vi "Update Values Buffer.vi"(8 "error in (no error)":errorcluster, 9 "buffer data":T1={"decimation"=0, "avg bandwidth"=0.0, "channels"=[], "byte order"=enum."little-endian", "buffer descriptor"={"buffer type"=enum."Engine", "plugin id"=0, "group id"=0, "transfer id"=0, "offset"=0, "length"=0}, "values channels"={"index"=0, "count"=0, "engine offset"=0}, "select start offset"=18446744073709551615, "select end offset"=0, "channel index"=-1} {"channels"."core"."string offset" format="%d bytes"; "avg bandwidth" format="%.0g bytes"}, 10 "buffer in":u8[](array[numeric]), 11 "values buffer in":u8[](array[numeric])) -> (0 "error out":errorcluster, 2 "buffer out":u8[](array[numeric]), 3 "values buffer out":u8[](array[numeric]))   [LabVIEW 2017, in "DSF Core.lvlib"]
uses:
  DSF Core.lvlib
  Buffer Reader/Buffer Data.ctl
  Typedefs/DSF Engine Channel Configuration.ctl
  Typedefs/Core Channel Configuration.ctl
  Typedefs/DSF Data Type.ctl
  Typedefs/DSF Settings Info.ctl
  Typedefs/DSF Version Info.ctl
  Typedefs/DSF Byte Order.ctl
  Classes/Thread/Data Server/DSF Buffer Subset Descriptor.ctl
  Typedefs/DSF Buffer Type.ctl
  Values Channels.ctl
  Classes/Framework/Framework.lvclass
  Classes/Configuration/Base/Channel/Channel Configuration.lvclass
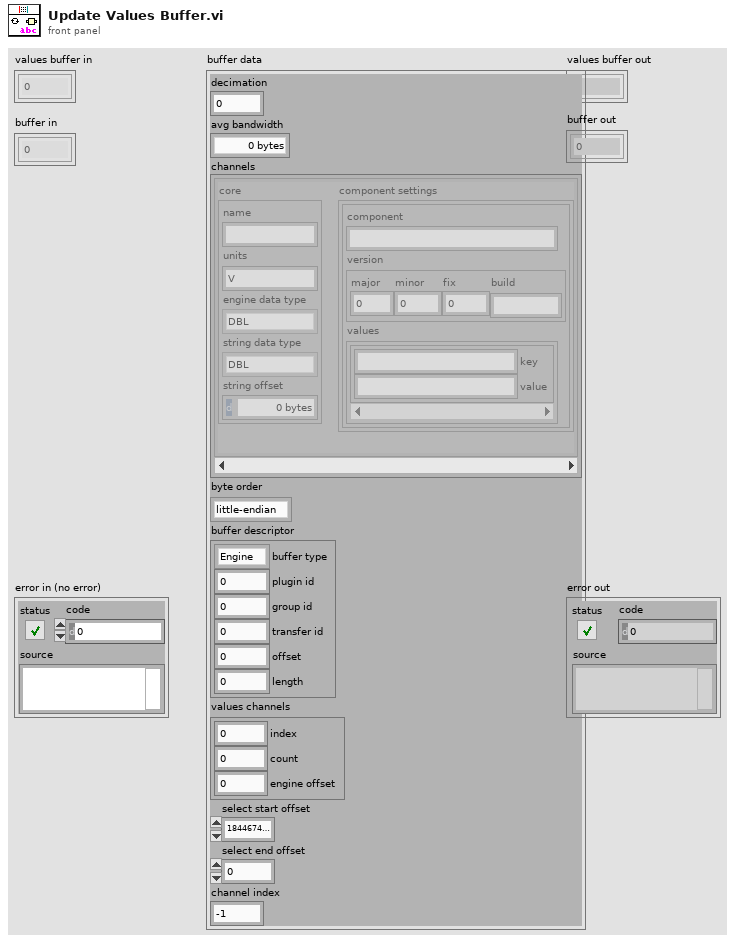
[diagram p1: front panel]
types:
  T1 = typedef "DSF Core.lvlib/Buffer Data.ctl" = cluster{"decimation":u64, "avg bandwidth":dbl, "channels":T2[], "byte order":T7, "buffer descriptor":T8, "values channels":T10, "select start offset":u64, "select end offset":u64, "channel index":i32}
  T2 = typedef "DSF Core.lvlib/DSF Engine Channel Configuration.ctl" = cluster{"core":T3, "component settings":T5[]}
  T3 = typedef "DSF Core.lvlib/Channel Configuration.lvclass/Core Channel Configuration.ctl" = cluster{"name":string, "units":string, "engine data type":T4, "string data type":T4, "string offset":u64}
  T4 = typedef "DSF Core.lvlib/DSF Data Type.ctl" = enum8{"Bool", "SGL", "DBL", "I8", "I16", "I32", "I64", "U8", "U16", "U32", "U64"}
  T5 = typedef "DSF Core.lvlib/DSF Settings Info.ctl" = cluster{"component":string, "version":T6, "values":cluster{"key":string, "value":string}[]}
  T6 = typedef "DSF Core.lvlib/DSF Version Info.ctl" = cluster{"major":u32, "minor":u32, "fix":u32, "build":string}
  T7 = typedef "DSF Core.lvlib/DSF Byte Order.ctl" = enum8{"big-endian", "little-endian"}
  T8 = typedef "DSF Core.lvlib/DSF Buffer Subset Descriptor.ctl" = cluster{"buffer type":T9, "plugin id":i32, "group id":i32, "transfer id":i32, "offset":u64, "length":i64}
  T9 = typedef "DSF Core.lvlib/DSF Buffer Type.ctl" = enum16{"Engine", "String"}
  T10 = typedef "DSF Core.lvlib/Values Channels.ctl" = cluster{"index":i32, "count":i32, "engine offset":u64}
  T11 = enum16{"big-endian, network order", "native, host order", "little-endian"}
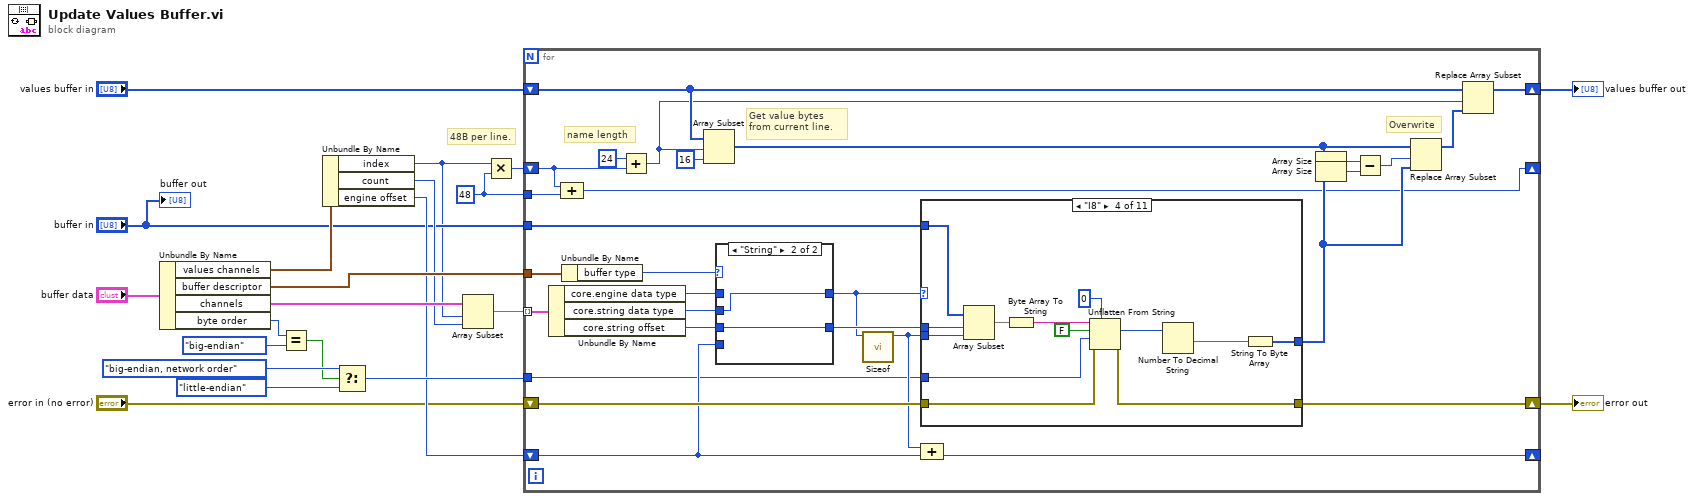
[diagram p0: block diagram]
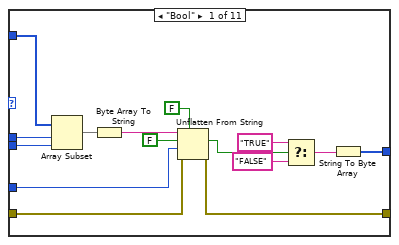
[diagram p3: hidden frame]
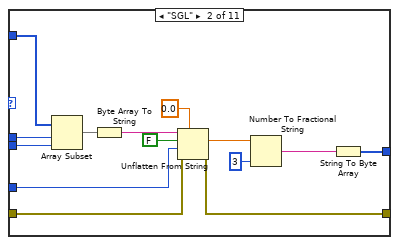
[diagram p4: hidden frame]
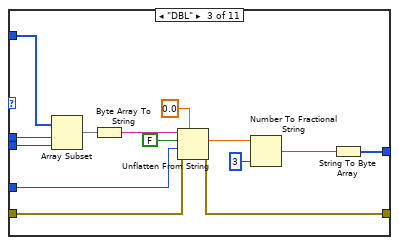
[diagram p5: hidden frame]
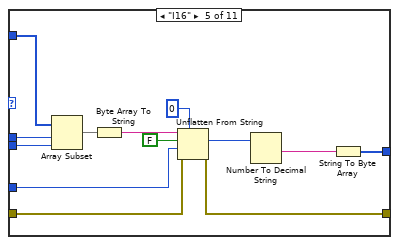
[diagram p6: hidden frame]
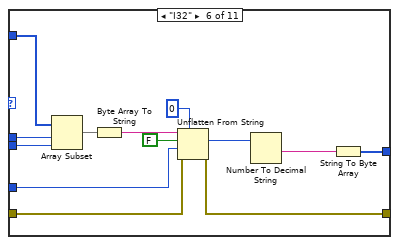
[diagram p7: hidden frame]
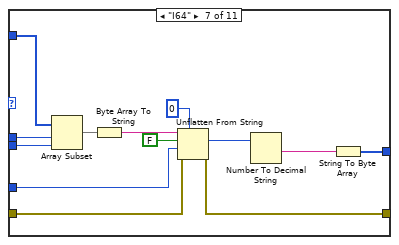
[diagram p8: hidden frame]
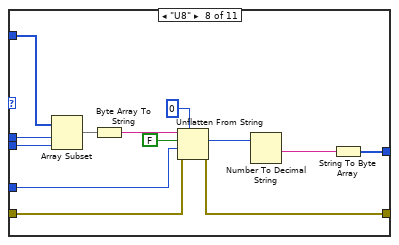
[diagram p9: hidden frame]
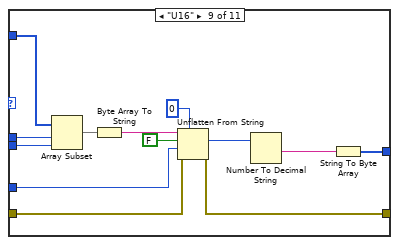
[diagram p10: hidden frame]
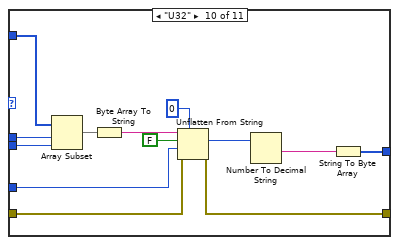
[diagram p11: hidden frame]
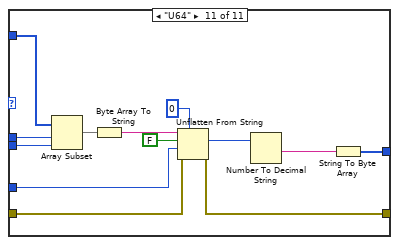
[diagram p12: hidden frame]
diagram:
  w1 = 48 ("x")
  # "48B per line."
  n1 = Unbundle By Name("buffer data") -> ("values channels"=w19:T10, "buffer descriptor"=w18:T8, "channels"=w17:T2[], "byte order"=w9:T7)
  n2 = Equal?(x=w9, y=DSF_Byte_Order."big-endian") -> (x = y?=w5:bool)
  n3 = Unbundle By Name(w19) -> ("index"=w2:i32, "count"=w10:i32, "engine offset"=w7:u64)
  n4 = Select(t=T11."big-endian, network order" ("byte order (0:big-endian, network order)"), s=w5, f=T11."little-endian") -> (s? t:f=w13:T11)
  n5 = Array Subset(array=w17, index=w2, length=w10) -> (w21:T2[])
  n6 = Multiply(x=w2, y=w1) -> (x*y=w3:i32)
  n7 = for {
    shift-right: [w25] -> w8
    shift-left: "error in (no error)" -> [w50]
    tunnel: w21 -> [w49] mode=indexing
    tunnel: w18 -> [w43]
    shift-right: [w44] -> _
    shift-left: w7 -> [w42]
    tunnel: w13 -> [w36]
    shift-right: [w40] -> w11
    shift-left: "values buffer in" -> [w41]
    tunnel: "buffer in" -> [w35]
    shift-right: [w26] -> _
    shift-left: w3 -> [w27]
    tunnel: w1 -> [w28]
    # "name length"
    # "Overwrite"
    # "Get value bytes from current line."
    n8 = Unbundle By Name(w49) -> ("core.engine data type"=w46:T4, "core.string data type"=w47:T4, "core.string offset"=w48:u64)
    n9 = Compound Arithmetic op=ADD(w27, w28) -> (w26:i32)
    n10 = Unbundle By Name(w43) -> ("buffer type"=w22:T9)
    n11 = Add(x=24, y=w27) -> (x+y=w37:i32)
    n12 = Array Subset(array=w41, index=w37, length=16) -> (w31:u8[])
    n13 = case shown="\"String\"" w22 {
      tunnel: w48 -> [_ w54]
      tunnel: [w51 w54] -> w24
      tunnel: w47 -> [_ w53]
      tunnel: w46 -> [w52 _]
      tunnel: w42 -> [w51 _]
      tunnel: [w52 w53] -> w23
      frame "Engine" {
      }
      frame "String" {
      }
    }
    n14 = call "Sizeof.vi"("data type"=w23) -> ("size in bytes"=w45:u64)  [unwired: 9 in, 1 out]
    n15 = case shown="\"I8\"" w23 {
      tunnel: w50 -> [w69 w83 w97 w110 w123 w136 w149 w162 w175 w188 w201]
      tunnel: [w68 w82 w96 w109 w122 w135 w148 w161 w174 w187 w200] -> w25
      tunnel: w24 -> [w61 w77 w91 w104 w117 w130 w143 w156 w169 w182 w195]
      tunnel: w45 -> [w62 w78 w92 w105 w118 w131 w144 w157 w170 w183 w196]
      tunnel: w36 -> [w60 w76 w90 w103 w116 w129 w142 w155 w168 w181 w194]
      tunnel: w35 -> [w59 w75 w89 w102 w115 w128 w141 w154 w167 w180 w193]
      tunnel: [w56 w73 w87 w100 w113 w126 w139 w152 w165 w178 w191] -> w29
      frame "Bool" {
        n16 = Array Subset(array=w59, index=w61, length=w62) -> (w58:u8[])
        n17 = Byte Array To String(unsigned byte array=w58) -> (string=w67:string)
        n18 = Unflatten From String(type=FALSE, binary string=w67, data includes array or string size? (T)=FALSE, byte order (0:big-endian, network order)=w60, error in (no error)=w69) -> (value=w55:bool, error out=w68:errorcluster)  [unwired: 1 out]
        n19 = Select(t="TRUE", s=w55, f="FALSE") -> (s? t:f=w57:string)
        n20 = String To Byte Array(string=w57) -> (unsigned byte array=w56:u8[])
      }
      frame "SGL" {
        n21 = Array Subset(array=w75, index=w77, length=w78) -> (w74:u8[])
        n22 = Byte Array To String(unsigned byte array=w74) -> (string=w81:string)
        n23 = Unflatten From String(type=sgl 0.0, binary string=w81, data includes array or string size? (T)=FALSE, byte order (0:big-endian, network order)=w76, error in (no error)=w83) -> (value=w71:sgl, error out=w82:errorcluster)  [unwired: 1 out]
        n24 = Number To Fractional String(number=w71, precision (6)=i16 3) -> (F-format string=w70:string)  [unwired: 2 in]
        n25 = String To Byte Array(string=w70) -> (unsigned byte array=w73:u8[])
      }
      frame "DBL" {
        n26 = Array Subset(array=w89, index=w91, length=w92) -> (w88:u8[])
        n27 = Byte Array To String(unsigned byte array=w88) -> (string=w95:string)
        n28 = Unflatten From String(type=0.0, binary string=w95, data includes array or string size? (T)=FALSE, byte order (0:big-endian, network order)=w90, error in (no error)=w97) -> (value=w85:dbl, error out=w96:errorcluster)  [unwired: 1 out]
        n29 = Number To Fractional String(number=w85, precision (6)=i16 3) -> (F-format string=w84:string)  [unwired: 2 in]
        n30 = String To Byte Array(string=w84) -> (unsigned byte array=w87:u8[])
      }
      frame "I8" {
        n31 = Array Subset(array=w102, index=w104, length=w105) -> (w101:u8[])
        n32 = Byte Array To String(unsigned byte array=w101) -> (string=w108:string)
        n33 = Unflatten From String(type=i8 0, binary string=w108, data includes array or string size? (T)=FALSE, byte order (0:big-endian, network order)=w103, error in (no error)=w110) -> (value=w99:i8, error out=w109:errorcluster)  [unwired: 1 out]
        n34 = Number To Decimal String(number=w99) -> (decimal integer string=w98:string)  [unwired: 1 in]
        n35 = String To Byte Array(string=w98) -> (unsigned byte array=w100:u8[])
      }
      frame "I16" {
        n36 = Array Subset(array=w115, index=w117, length=w118) -> (w114:u8[])
        n37 = Byte Array To String(unsigned byte array=w114) -> (string=w121:string)
        n38 = Unflatten From String(type=i16 0, binary string=w121, data includes array or string size? (T)=FALSE, byte order (0:big-endian, network order)=w116, error in (no error)=w123) -> (value=w112:i16, error out=w122:errorcluster)  [unwired: 1 out]
        n39 = Number To Decimal String(number=w112) -> (decimal integer string=w111:string)  [unwired: 1 in]
        n40 = String To Byte Array(string=w111) -> (unsigned byte array=w113:u8[])
      }
      frame "I32" {
        n41 = Array Subset(array=w128, index=w130, length=w131) -> (w127:u8[])
        n42 = Byte Array To String(unsigned byte array=w127) -> (string=w134:string)
        n43 = Unflatten From String(type=0, binary string=w134, data includes array or string size? (T)=FALSE, byte order (0:big-endian, network order)=w129, error in (no error)=w136) -> (value=w125:i32, error out=w135:errorcluster)  [unwired: 1 out]
        n44 = Number To Decimal String(number=w125) -> (decimal integer string=w124:string)  [unwired: 1 in]
        n45 = String To Byte Array(string=w124) -> (unsigned byte array=w126:u8[])
      }
      frame "I64" {
        n46 = Array Subset(array=w141, index=w143, length=w144) -> (w140:u8[])
        n47 = Byte Array To String(unsigned byte array=w140) -> (string=w147:string)
        n48 = Unflatten From String(type=i64 0, binary string=w147, data includes array or string size? (T)=FALSE, byte order (0:big-endian, network order)=w142, error in (no error)=w149) -> (value=w138:i64, error out=w148:errorcluster)  [unwired: 1 out]
        n49 = Number To Decimal String(number=w138) -> (decimal integer string=w137:string)  [unwired: 1 in]
        n50 = String To Byte Array(string=w137) -> (unsigned byte array=w139:u8[])
      }
      frame "U8" {
        n51 = Array Subset(array=w154, index=w156, length=w157) -> (w153:u8[])
        n52 = Byte Array To String(unsigned byte array=w153) -> (string=w160:string)
        n53 = Unflatten From String(type=u8 0, binary string=w160, data includes array or string size? (T)=FALSE, byte order (0:big-endian, network order)=w155, error in (no error)=w162) -> (value=w151:u8, error out=w161:errorcluster)  [unwired: 1 out]
        n54 = Number To Decimal String(number=w151) -> (decimal integer string=w150:string)  [unwired: 1 in]
        n55 = String To Byte Array(string=w150) -> (unsigned byte array=w152:u8[])
      }
      frame "U16" {
        n56 = Array Subset(array=w167, index=w169, length=w170) -> (w166:u8[])
        n57 = Byte Array To String(unsigned byte array=w166) -> (string=w173:string)
        n58 = Unflatten From String(type=u16 0, binary string=w173, data includes array or string size? (T)=FALSE, byte order (0:big-endian, network order)=w168, error in (no error)=w175) -> (value=w164:u16, error out=w174:errorcluster)  [unwired: 1 out]
        n59 = Number To Decimal String(number=w164) -> (decimal integer string=w163:string)  [unwired: 1 in]
        n60 = String To Byte Array(string=w163) -> (unsigned byte array=w165:u8[])
      }
      frame "U32" {
        n61 = Array Subset(array=w180, index=w182, length=w183) -> (w179:u8[])
        n62 = Byte Array To String(unsigned byte array=w179) -> (string=w186:string)
        n63 = Unflatten From String(type=u32 0, binary string=w186, data includes array or string size? (T)=FALSE, byte order (0:big-endian, network order)=w181, error in (no error)=w188) -> (value=w177:u32, error out=w187:errorcluster)  [unwired: 1 out]
        n64 = Number To Decimal String(number=w177) -> (decimal integer string=w176:string)  [unwired: 1 in]
        n65 = String To Byte Array(string=w176) -> (unsigned byte array=w178:u8[])
      }
      frame "U64" {
        n66 = Array Subset(array=w193, index=w195, length=w196) -> (w192:u8[])
        n67 = Byte Array To String(unsigned byte array=w192) -> (string=w199:string)
        n68 = Unflatten From String(type=u64 0, binary string=w199, data includes array or string size? (T)=FALSE, byte order (0:big-endian, network order)=w194, error in (no error)=w201) -> (value=w190:u64, error out=w200:errorcluster)  [unwired: 1 out]
        n69 = Number To Decimal String(number=w190) -> (decimal integer string=w189:string)  [unwired: 1 in]
        n70 = String To Byte Array(string=w189) -> (unsigned byte array=w191:u8[])
      }
    }
    n71 = Compound Arithmetic op=ADD(w45, w42) -> (w44:u64)
    n72 = Array Size(array=w31) -> (size(s)=w34:i32)
    n73 = Array Size(array=w29) -> (size(s)=w33:i32)
    n74 = Subtract(x=w34, y=w33) -> (x-y=w32:i32)
    n75 = Replace Array Subset(array=w31, new element=w29, index=w32) -> (w30:u8[])
    n76 = Replace Array Subset(array=w41, new element=w30, index=w37) -> (w40:u8[])
  }
  "values buffer out" <- w11
  "error out" <- w8
  "buffer out" <- "buffer in"
